vi "Init.vi"(8 "error in":errorcluster, 11 "DAQmx Base Configure Strategy in":refnum<class "DAQmx Base Configure Strategy.lvclass">) -> (0 "error out":errorcluster, 3 "DAQmx Base Configure Strategy out":refnum<class "DAQmx Base Configure Strategy.lvclass">)   [LabVIEW 2024, in "DAQmx Base Configure Strategy.lvclass"]
uses:
  DAQmx Base Configure Strategy.lvclass
  DAQmx Base Configure Strategy.lvclass/DAQmx Base Configure Strategy.ctl
  Source/Interfaces/IConfiguration/IConfiguration.lvclass
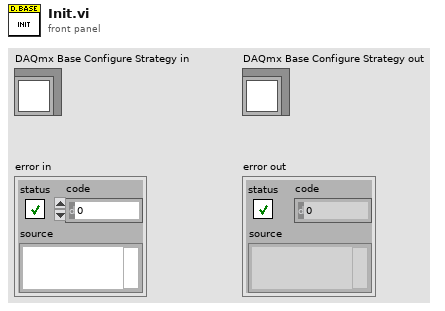
[diagram p1: front panel]
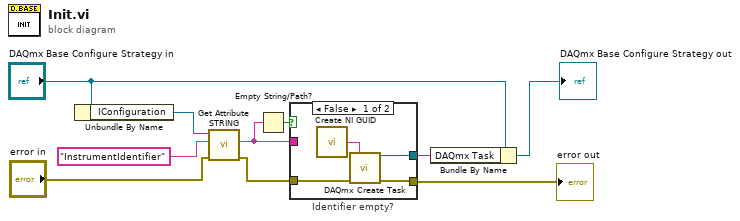
[diagram p0: block diagram]
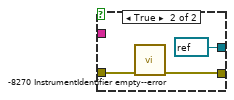
[diagram p2: hidden frame]
diagram:
  n1 = Unbundle By Name("DAQmx Base Configure Strategy in") -> ("IConfiguration"=w8:refnum<class "IConfiguration.lvclass">)
  n2 = call-dynamic "Get Attribute STRING.vi"("error in"="error in", "Attribute"="InstrumentIdentifier", "IConfiguration in"=w8) -> ("error out"=w3:errorcluster, "Value"=w1:string)  [unwired: 6 in, 1 out]
  n3 = Empty String/Path?(string/path=w1) -> (empty?=w10:bool)
  n4 = case "Identifier empty?" shown="False" w10 {
    tunnel: w3 -> [w11 w16]
    tunnel: [w14 w15] -> w2
    tunnel: [w12 refnum<k21> refnum ("task out")] -> w9
    tunnel: w1 -> [_ _]
    frame False {
      n5 = call <vilib>:"Create NI GUID.vi"() -> ("NI GUID"=w13:string)
      n6 = call <vilib>:"DAQmx Create Task.vi"("new task name"=w13, "error in"=w11) -> ("task out"=w12:refnum<k21>, "error out"=w14:errorcluster)  [unwired: 12 in]
    }
    frame True {
      n7 = call "-8270 InstrumentIdentifier empty--error.vi"("error in"=w16) -> ("error out"=w15:errorcluster)  [unwired: 10 in]
    }
  }
  "error out" <- w2
  n8 = Bundle By Name(cluster="DAQmx Base Configure Strategy in", "DAQmx Task"=w9) -> (→"DAQmx Base Configure Strategy out":refnum<class "DAQmx Base Configure Strategy.lvclass">)
